vi "data_processing_loop.vi"(8 "error in (no error)":errorcluster, 10 "Notifiers":T1, 11 "Message Queues":T2) -> (0 "error out":errorcluster)   [LabVIEW 2017, in "data_processing.lvlib"]
uses:
  data_processing.lvlib
  support/Message Queue/All Message Queues.ctl
  support/Message Queue/Message Cluster.ctl
  support/Notifiers/Notifiers.ctl
  dataframe/DataFrame.lvclass
  <vilib>/Utility/error.llb/Error Cluster From Error Code.vi
  <vilib>/ErrorRing/Error Ring.xnode
  support/Message Queue/Message Queue.lvlib
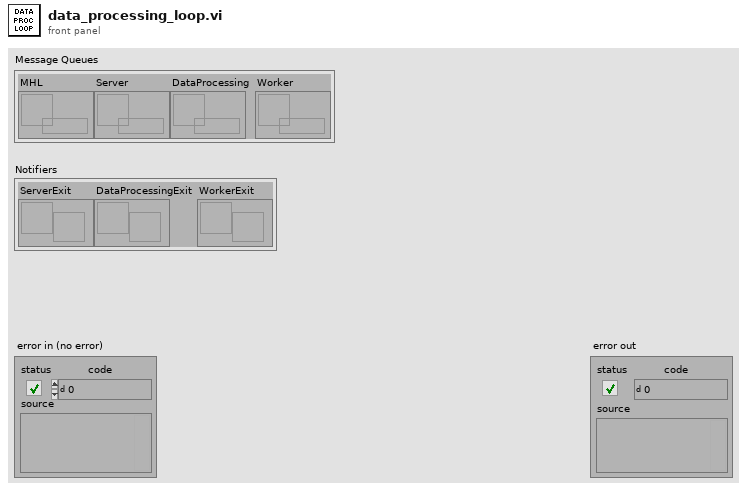
[diagram p1: front panel]
types:
  T1 = typedef "Notifiers.ctl" = cluster{"ServerExit":refnum<notifier>, "DataProcessingExit":refnum<notifier>, "WorkerExit":refnum<notifier>}
  T2 = typedef "Message Queue.lvlib/All Message Queues.ctl" = cluster{"MHL":refnum<queue>, "Server":refnum<queue>, "DataProcessing":refnum<queue>, "Worker":refnum<queue>}
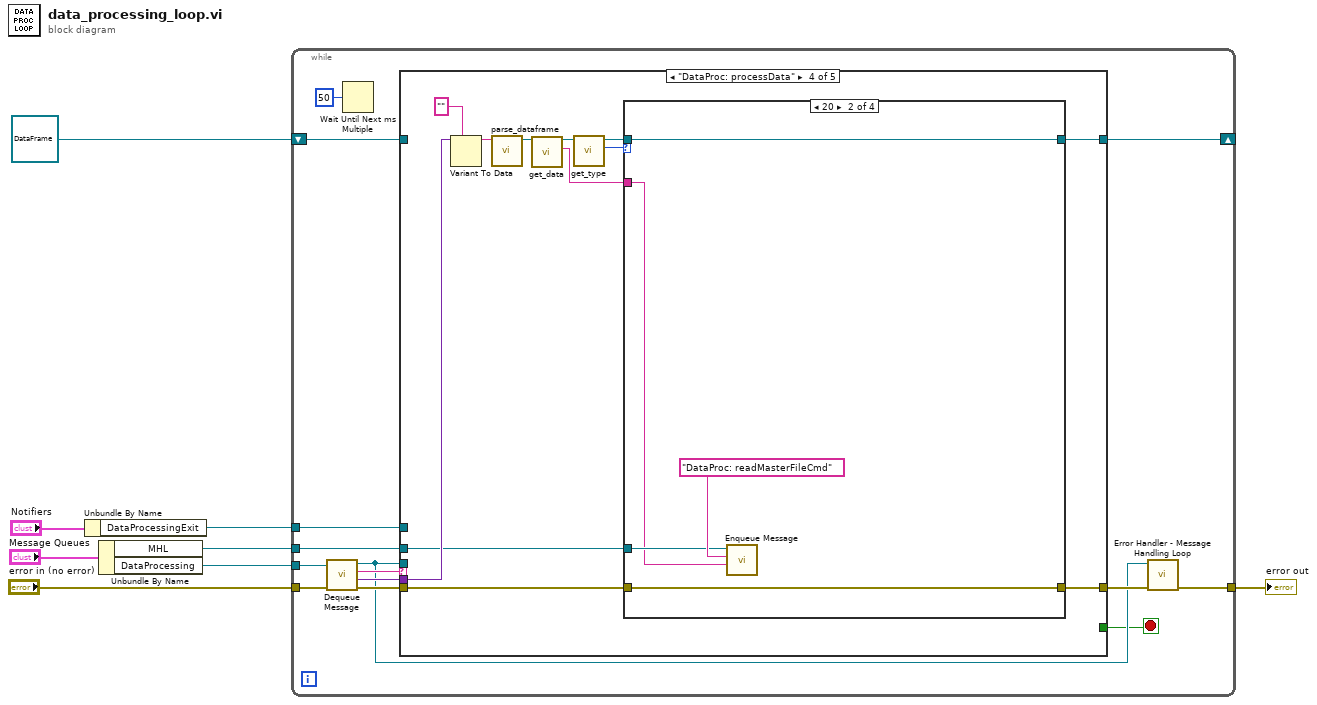
[diagram p0: block diagram]
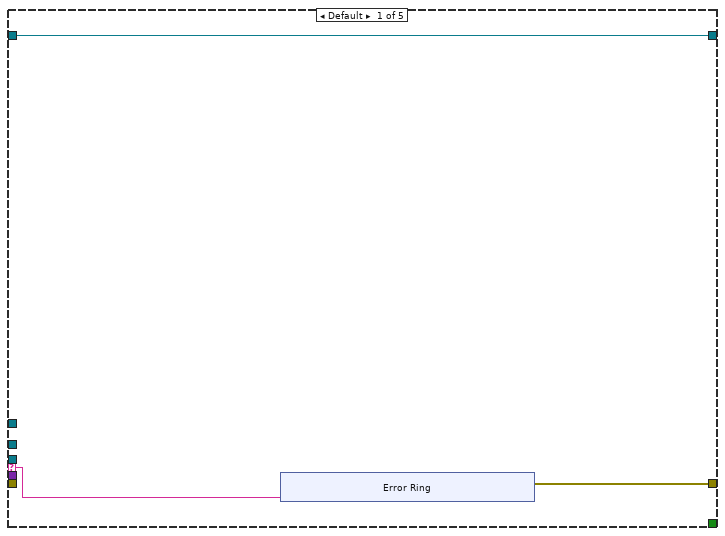
[diagram p2: hidden frame]
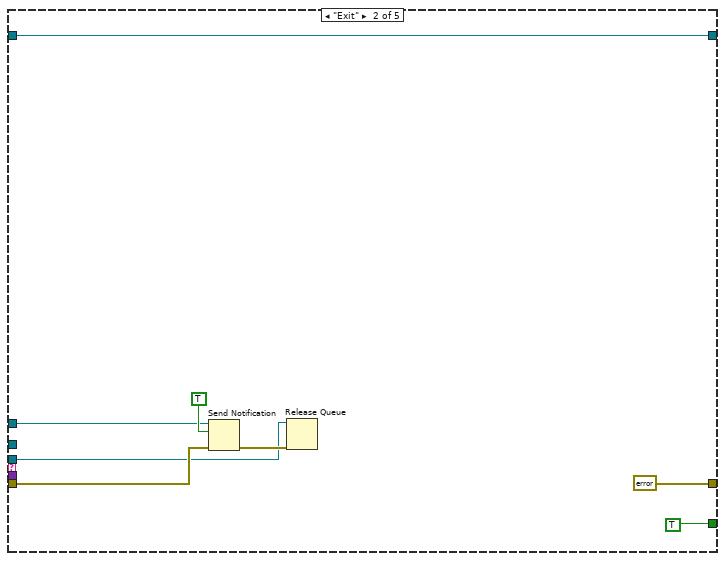
[diagram p3: hidden frame]
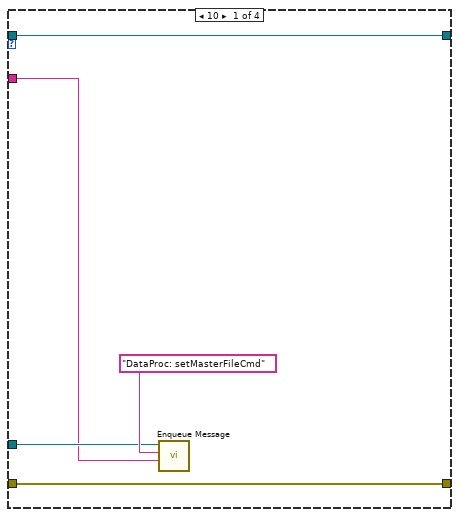
[diagram p5: hidden frame]
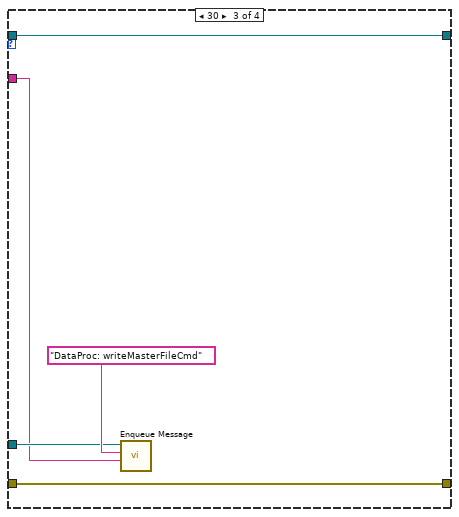
[diagram p6: hidden frame]
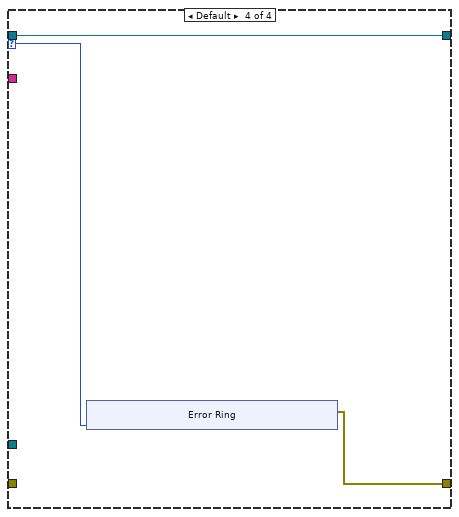
[diagram p7: hidden frame]
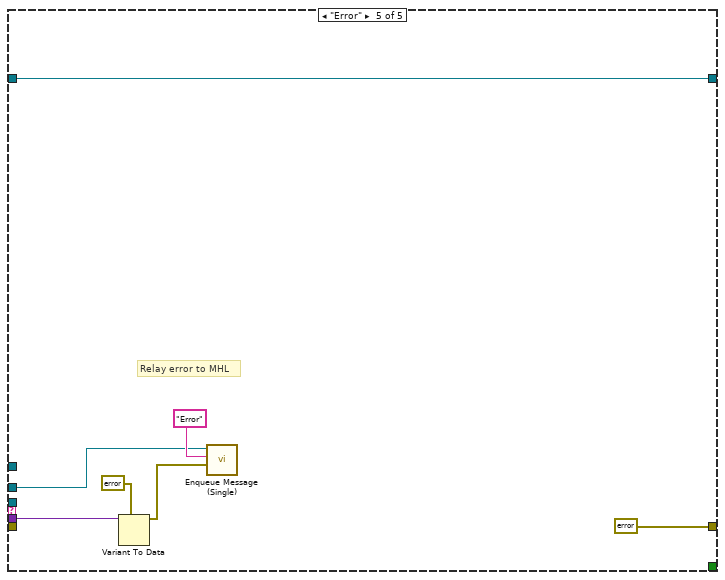
[diagram p8: hidden frame]
diagram:
  n1 = Unbundle By Name("Notifiers") -> ("DataProcessingExit"=w4:refnum<notifier>)
  n2 = Unbundle By Name("Message Queues") -> ("MHL"=w7:refnum<queue>, "DataProcessing"=w6:refnum<queue>)
  n3 = while {
    tunnel: w7 -> [w13]
    tunnel: w6 -> [w22]
    tunnel: w4 -> [w9]
    tunnel: "error in (no error)" -> [w21]
    tunnel: [w15] -> w2
    shift-right: [w10] -> _
    shift-left: refnum<class "DataFrame.lvclass"> refnum ("DataFrame.lvclass") -> [w11]
    stop <- w14 stop-if-true
    n4 = call "Dequeue Message.vi"("error in (no error)"=w21, "Message Queue"=w22) -> ("error out"=w19:errorcluster, "Message Data"=w17:variant, "Message"=w18:string, "dup Message Queue"=w16:refnum<queue>)  [unwired: 6 in]
    n5 = Wait Until Next ms Multiple(millisecond multiple=u32 50) -> ()  [unwired: 1 out]
    n6 = case shown="\"DataProc: processData\"" w18 {
      selector: w18 -> [w25 _ _ _ _]
      tunnel: [w24 errorcluster {"status"=FALSE, "code"=0, "source"=""} ("error constant") w42 w50 errorcluster {"status"=FALSE, "code"=0, "source"=""} ("error constant")] -> w20
      tunnel: w19 -> [_ w35 w42 w51 _]
      tunnel: w17 -> [_ _ _ w54 w82]
      tunnel: w16 -> [_ w34 _ _ _]
      tunnel: [_ TRUE _ _ _] -> w14
      tunnel: w13 -> [_ _ _ w47 w84]
      tunnel: w11 -> [w23 w39 w41 _ w83]
      tunnel: [w23 w39 w41 w48 w83] -> w10
      tunnel: w9 -> [_ w37 _ _ _]
      frame Default {
        n7 = xnode "Error Ring"("parameter 0"=w25) -> ("error out"=w24:errorcluster)
      }
      frame "Exit" {
        n8 = Send Notification(notification=TRUE, notifier=w37, error in (no error)=w35) -> (error out=w36:errorcluster)  [unwired: 1 out]
        n9 = Release Queue(queue=w34, error in (no error)=w36) -> ()  [unwired: 1 in, 3 out]
      }
      frame "Initialize" {
      }
      frame "DataProc: processData" {
        n10 = Variant To Data(type="", Variant=w54) -> (data=w52:string)  [unwired: 1 in, 1 out]
        n11 = call "parse_dataframe.vi"("dataframe"=w52) -> ("DataFrame.lvclass"=w45:refnum<class "DataFrame.lvclass">)  [unwired: 10 in]
        n12 = call "get_data.vi"("DataFrame in"=w45) -> ("data"=w43:string, "DataFrame out"=w44:refnum<class "DataFrame.lvclass">)  [unwired: 8 in, 1 out]
        n13 = call "get_type.vi"("DataFrame in"=w44) -> ("type"=w46:u8, "DataFrame out"=w49:refnum<class "DataFrame.lvclass">)  [unwired: 8 in, 1 out]
        n14 = case shown="20" w46 {
          selector: w46 -> [_ _ _ w70]
          tunnel: w51 -> [w59 w64 w69 _]
          tunnel: [w59 w64 w69 w71] -> w50
          tunnel: w49 -> [w58 w63 w68 w72]
          tunnel: [w58 w63 w68 w72] -> w48
          tunnel: w47 -> [w56 w61 w66 _]
          tunnel: w43 -> [w55 w60 w65 _]
          frame 10 {
            n15 = call-poly "Enqueue Message.vi"("Message Data"=w55, "Message"="DataProc: setMasterFileCmd", "Message Queue"=w56) -> ()  [unwired: 7 in, 2 out]
          }
          frame 20 {
            n16 = call-poly "Enqueue Message.vi"("Message Data"=w60, "Message"="DataProc: readMasterFileCmd", "Message Queue"=w61) -> ()  [unwired: 7 in, 2 out]
          }
          frame 30 {
            n17 = call-poly "Enqueue Message.vi"("Message Data"=w65, "Message"="DataProc: writeMasterFileCmd", "Message Queue"=w66) -> ()  [unwired: 7 in, 2 out]
          }
          frame Default {
            n18 = xnode "Error Ring"("parameter 0"=w70) -> ("error out"=w71:errorcluster)
          }
        }
      }
      frame "Error" {
        # "Relay error to MHL"
        n19 = Variant To Data(type=errorcluster {"status"=FALSE, "code"=0, "source"=""} ("error constant"), Variant=w82) -> (data=w80:errorcluster)  [unwired: 1 in, 1 out]
        n20 = call "Enqueue Message (Single).vi"("Message Data"=w80, "Message"="Error", "Message Queue"=w84) -> ()  [unwired: 7 in, 2 out]
      }
    }
    n21 = call "Error Handler - Message Handling Loop.vi"("error in (no error)"=w20, "Message Queue"=w16) -> ("dup error in"=w15:errorcluster)  [unwired: 8 in, 1 out]
  }
  "error out" <- w2
